vi "get video info.vi"(8 "error in":errorcluster, 11 "Path":path) -> (0 "error out":errorcluster, 1 "Valid?":bool, 3 "video info":T1 {"date" format="%<%x>T"})   [LabVIEW 2023, in "File Classes.lvlib" / "Video File.lvclass"]
uses:
  Video File.lvclass
  Controls/video exif info cluster.ctl
  File Classes.lvlib
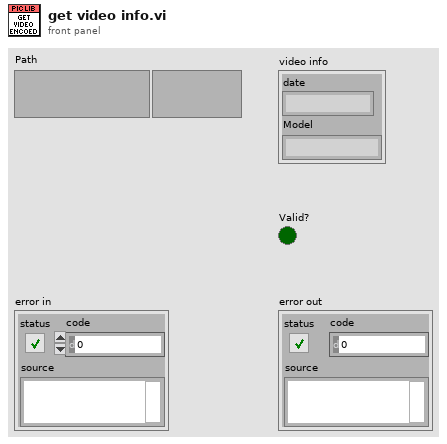
[diagram p1: front panel]
types:
  T1 = typedef "File Classes.lvlib/video exif info cluster.ctl" = cluster{"date":timestamp, "Model":string}
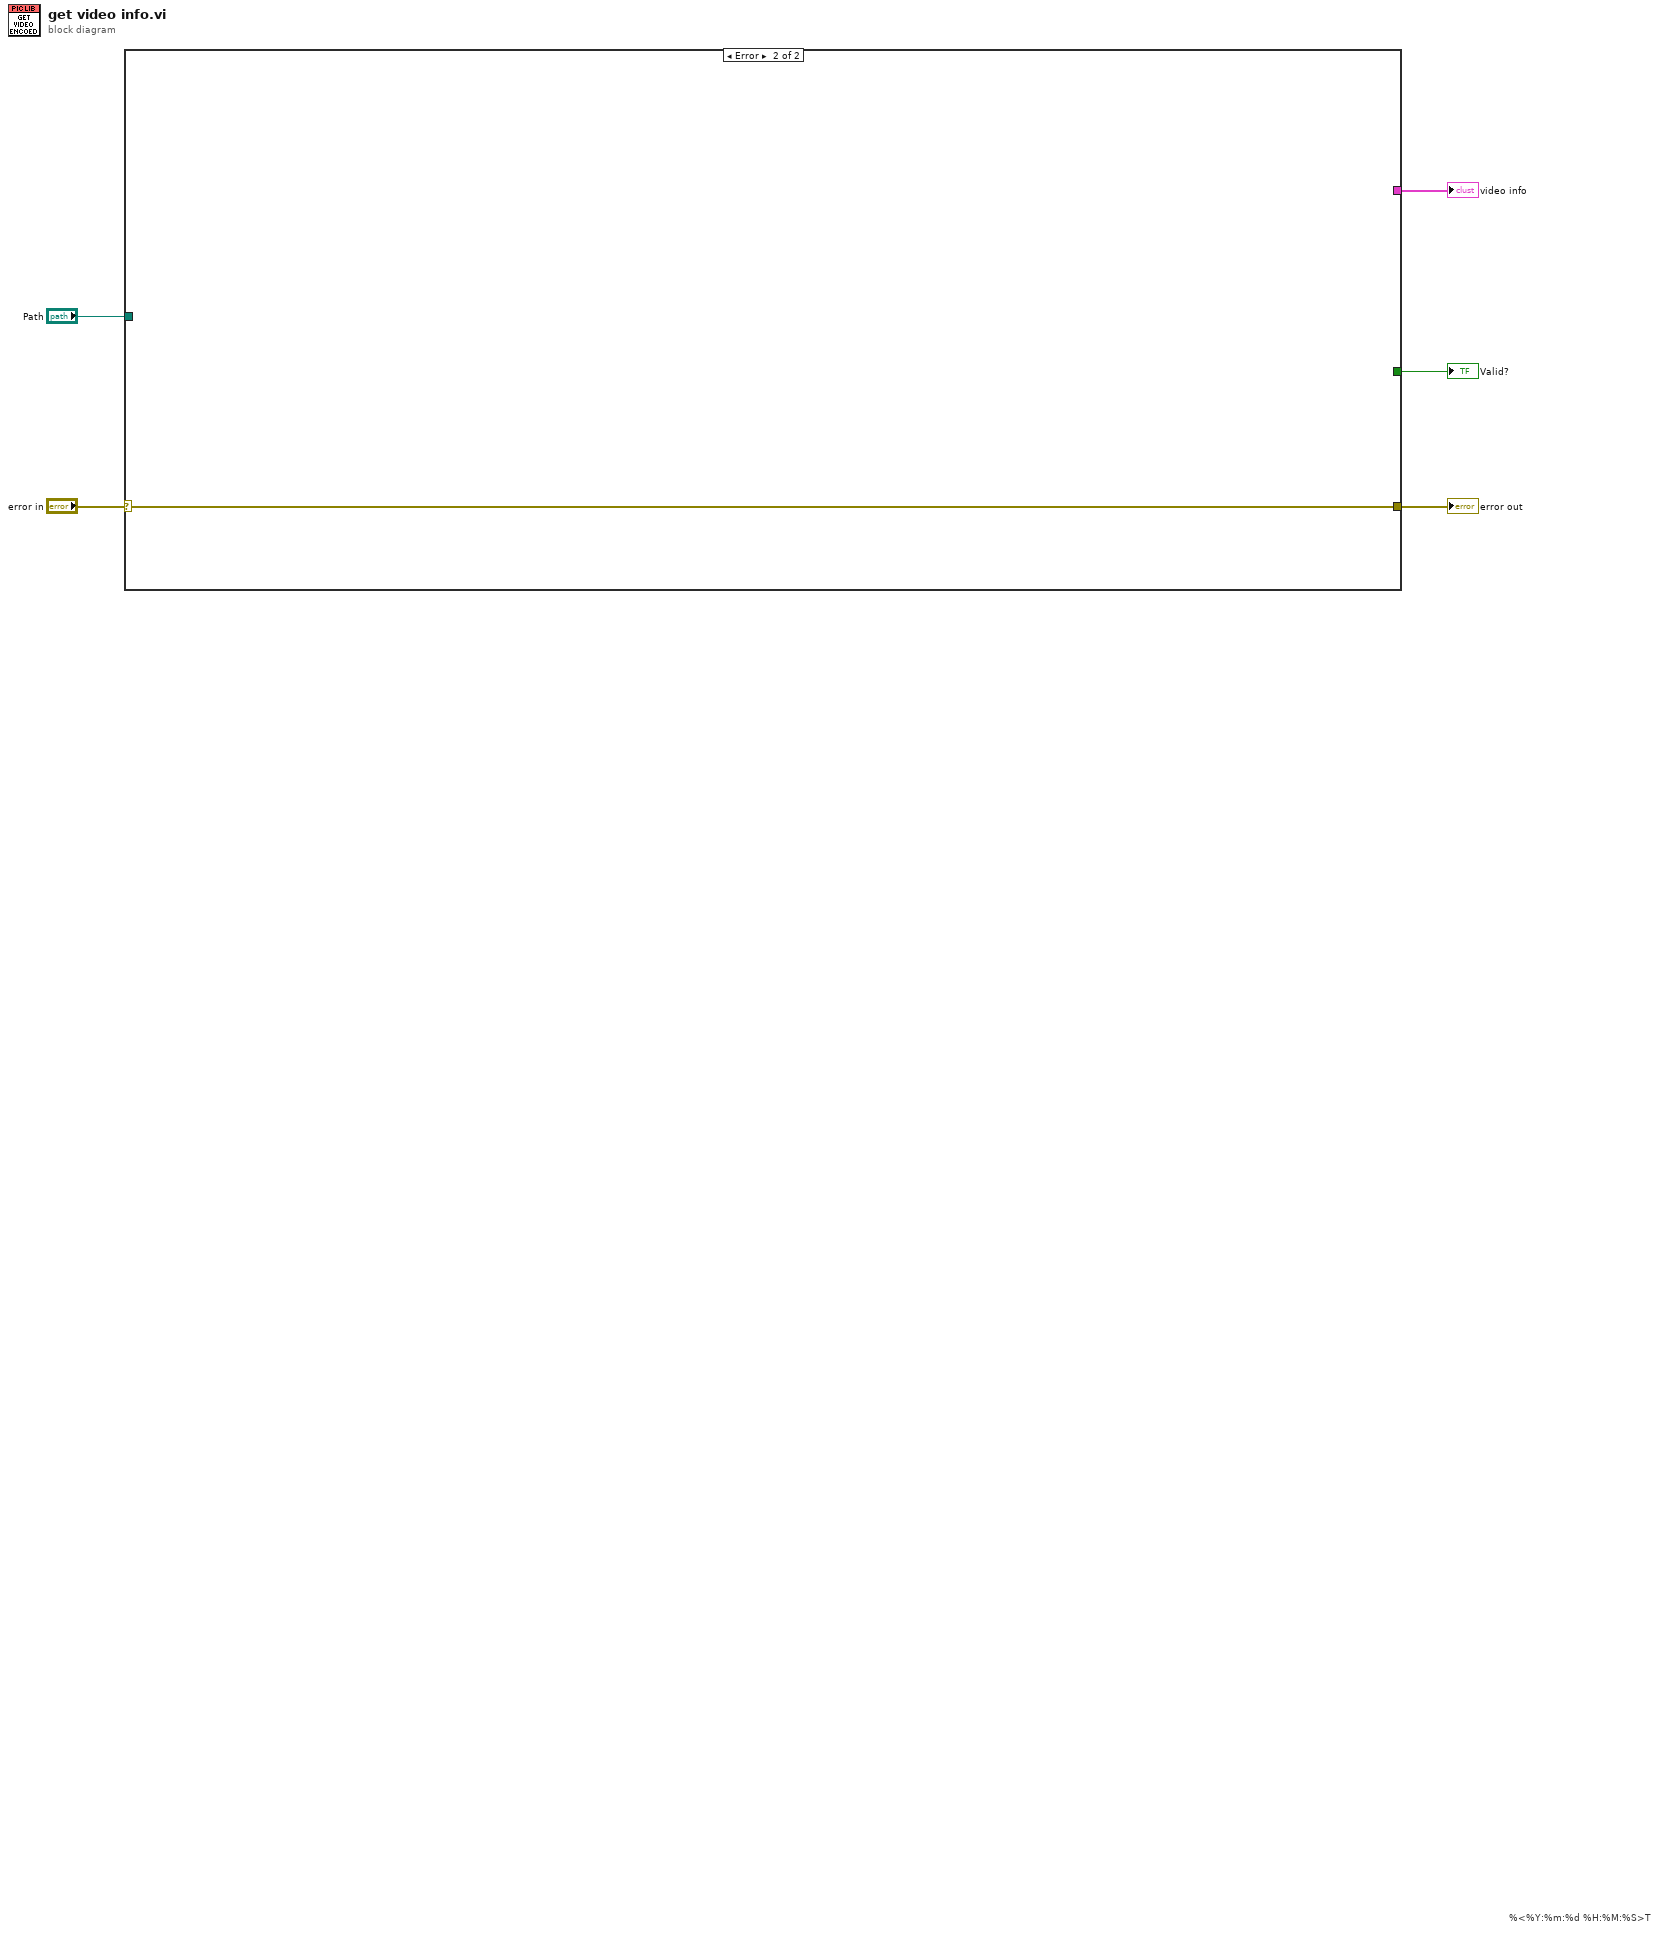
[diagram p0: block diagram]
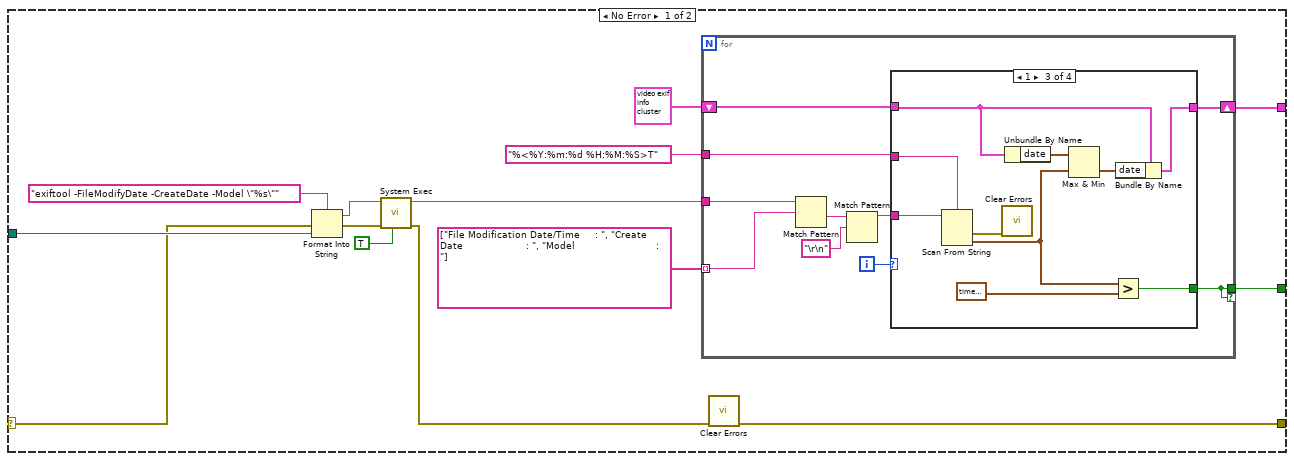
[diagram p2: hidden frame]
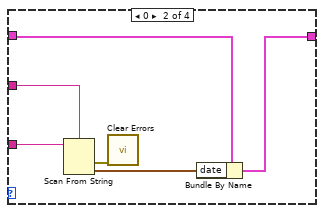
[diagram p4: hidden frame]
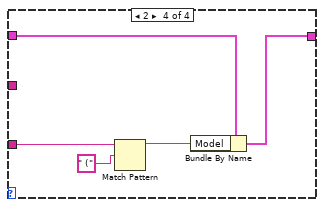
[diagram p5: hidden frame]
diagram:
  # "%<%Y:%m:%d %H:%M:%S>T"
  n1 = case shown="Error" "error in" {
    selector: "error in" -> [w14 w52]
    tunnel: "Path" -> [w18 _]
    tunnel: [w9 _] -> w3
    tunnel: [w6 w52] -> w2
    tunnel: [w7 _] -> w1
    frame No Error {
      n2 = Format Into String(format string="exiftool -FileModifyDate -CreateDate -Model \"%s\"" ("command line"), error in=w14, w18) -> (resulting string=w16:string, error out=w15:errorcluster)  [unwired: 1 in]
      n3 = call <vilib>:"System Exec.vi"("run minimized? (F)"=TRUE, "error in (no error)"=w15, "command line"=w16) -> ("error out"=w8:errorcluster, "standard output"=w11:string)  [unwired: 5 in, 2 out]
      n4 = for {
        tunnel: w11 -> [w29]
        tunnel: string[] ["File Modification Date/Time     : ", "Create Date                     : ", "Model                           : "] -> [w28] mode=indexing
        shift-right: [w22] -> w7
        shift-left: T1 {"date"=timestamp(0 s since 1904-01-01), "Model"=""} ("video info") -> [w23]
        tunnel: [w21] -> w9 if=w21
        tunnel: "%<%Y:%m:%d %H:%M:%S>T" ("format string") -> [w20]
        i -> [w24]
        n5 = Match Pattern(string=w29, regular expression=w28) -> (after substring=w27:string)  [unwired: 1 in, 3 out]
        n6 = Match Pattern(string=w27, regular expression="\r\n") -> (before substring=w25:string)  [unwired: 1 in, 3 out]
        n7 = case shown="1" w24 {
          tunnel: w25 -> [_ w36 w46 w47]
          tunnel: w20 -> [_ w35 w45 _]
          tunnel: w23 -> [w30 w32 w42 w50]
          tunnel: [w30 w33 w43 w51] -> w22
          tunnel: [_ _ w40 _] -> w21
          frame Default {
          }
          frame 0 {
            n8 = Scan From String(format string=w35, input string=w36) -> (error out=w34:errorcluster, output 1=w31:timestamp)  [unwired: 3 in, 2 out]
            n9 = call <vilib>:"Clear Errors.vi"("error in (no error)"=w34) -> ()  [unwired: 5 in, 2 out]
            n10 = Bundle By Name(cluster=w32, "date"=w31) -> (w33:T1)
          }
          frame 1 {
            n11 = Scan From String(format string=w45, input string=w46) -> (error out=w44:errorcluster, output 1=w38:timestamp)  [unwired: 3 in, 2 out]
            n12 = call <vilib>:"Clear Errors.vi"("error in (no error)"=w44) -> ()  [unwired: 5 in, 2 out]
            n13 = Unbundle By Name(w42) -> ("date"=w39:timestamp)
            n14 = Max & Min(x=w39, y=w38) -> (min(x,y)=w37:timestamp)  [unwired: 1 out]
            n15 = Greater?(x=w38, y=timestamp(2714023800 s since 1904-01-01) ("output 1")) -> (0:w40:bool)
            n16 = Bundle By Name(cluster=w42, "date"=w37) -> (w43:T1)
          }
          frame 2 {
            n17 = Match Pattern(string=w47, regular expression=" (") -> (before substring=w48:string)  [unwired: 1 in, 3 out]
            n18 = Bundle By Name(cluster=w50, "Model"=w48) -> (w51:T1)
          }
        }
      }
      n19 = call <vilib>:"Clear Errors.vi"("error in (no error)"=w8) -> ("error out"=w6:errorcluster)  [unwired: 5 in, 1 out]
    }
    frame Error {
    }
  }
  "error out" <- w2
  "Valid?" <- w3
  "video info" <- w1
